vi "Ramp15_test.vi"() -> ()   [LabVIEW 2016]
uses:
  BERTTA.dll
panel:
  in  "port":i32
  out "target_reached":dbl
  out "reset_out":dbl
  out "T control":dbl
  in  "time_set":dbl
  out "params":dbl[](array[numeric])
  in  "manual":i32
  in  "enable":i32
  in  "reset":i32
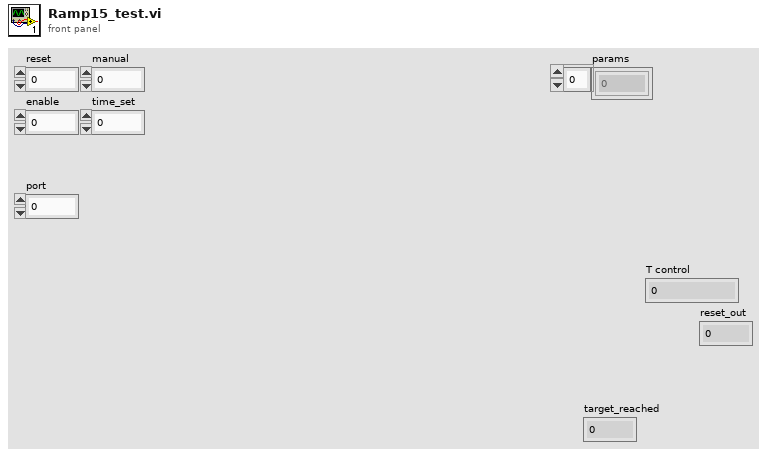
[diagram p1: front panel]
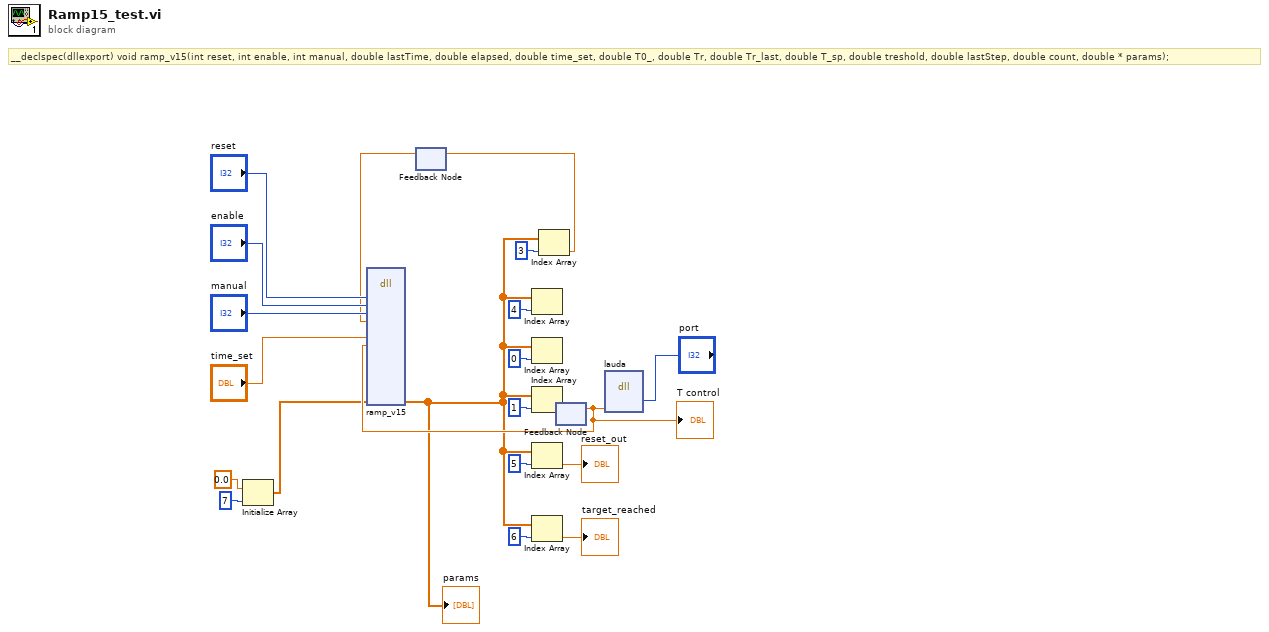
[diagram p0: block diagram]
diagram:
  # "__declspec(dllexport) void ramp_v15(int reset, int enable, int manual, double lastTime, double elapsed, double time_set, double T0_, double Tr, double Tr_last, double T_sp, double treshold, double lastStep, double count, double * params);"
  n1 = Initialize Array(0.0 ("element"), 7 ("dimension size")) -> (w5:dbl[])
  n2 = feedback #1() -> (w1:dbl)  [unwired: 1 in]
  n3 = feedback #2() -> (w8:dbl)  [unwired: 1 in]
  "T control" <- w8
  n4 = dll-call lib="C:/Users/shresplab/OneDrive - Kemira Oyj/Documents/GitHub/Bertta/BERTTA/x64/Debug/BERTTA.dll" fn="ramp_v15"("reset"="reset", "enable"="enable", "manual"="manual", "lastTime"=w1, "time_set"="time_set", "T0_"=w8, "params"=w5) -> ("params"=w3:dbl[])  [unwired: 24 in, 2 out]
  "params" <- w3
  n5 = Index Array(array=w3, index=4) -> ()  [unwired: 1 out]
  n6 = Index Array(array=w3, index=0) -> ()  [unwired: 1 out]
  n7 = Index Array(array=w3, index=1) -> (element=w9:dbl)
  n8 = Index Array(array=w3, index=5) -> (element=→"reset_out":dbl)
  n9 = Index Array(array=w3, index=6) -> (element=→"target_reached":dbl)
  n10 = Index Array(array=w3, index=3) -> (element=w2:dbl)
  n11 = feedback-in #1(w2) -> ()
  n12 = feedback-in #2(w9) -> ()
  n13 = dll-call lib="C:/Users/shresplab/OneDrive - Kemira Oyj/Documents/GitHub/Bertta/BERTTA/x64/Debug/BERTTA.dll" fn="lauda"("port"="port", "set_temp"=w8) -> ()  [unwired: 6 in, 2 out]
